vi "SHAPE_readTrainingData.vi"(8 "error in (no error)":errorcluster, 9 "ControlRefs":T1, 10 "NumberOfChannels":i32, 11 "BandGlobalOpt in":refnum<class "Shapelets Search GA.lvclass">) -> (0 "error out":errorcluster, 2 "TimeSeriesLength":i32, 3 "BandGlobalOpt out":refnum<class "Shapelets Search GA.lvclass">)   [LabVIEW 2016, in "Shapelets Search (GA).lvlib" / "Shapelets Search GA.lvclass"]
uses:
  Shapelets Search GA.lvclass
  Shapelets Search GA.lvclass/Shapelets Search GA.ctl
  <vilib>/xml/Load XML File.vi
  <vilib>/xml/Close Reference(Node).vi
  _XML_EEG_Features/XML_EEG_Features.lvlib
  <vilib>/xml/NI_XML.lvlib
panel:
  # "This VI is a part of BCI Design library, http://www.ru-bci.org \nCopyright © 2020, Sotnikov Peter, All rights reserved. License: CC BY-NC 4.0"
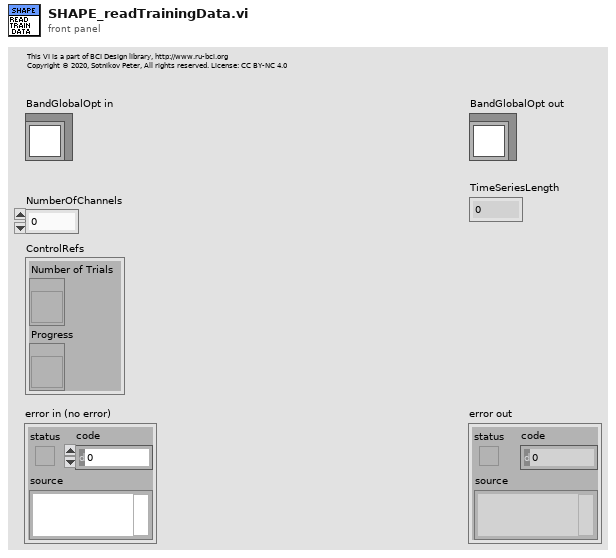
[diagram p1: front panel]
types:
  T1 = cluster{"Number of Trials":refnum<vi>, "Progress":refnum<vi>}
  T2 = typedef "XML_EEG_Features.lvlib/XML_FF_Header.ctl" = cluster{"NumberOfTrials":i32, "NumberOfClasses":i32, "FeatureVectorLength":i32, "FeatureExtractionMethod":string}
  T3 = typedef "XML_EEG_Features.lvlib/XML_FF_Trial.ctl" = cluster{"ClassLabel":string, "FeatureVector":dbl[]}
  T4 = cluster{"ClassLabel":string, "FeatureVector":dbl[][]}
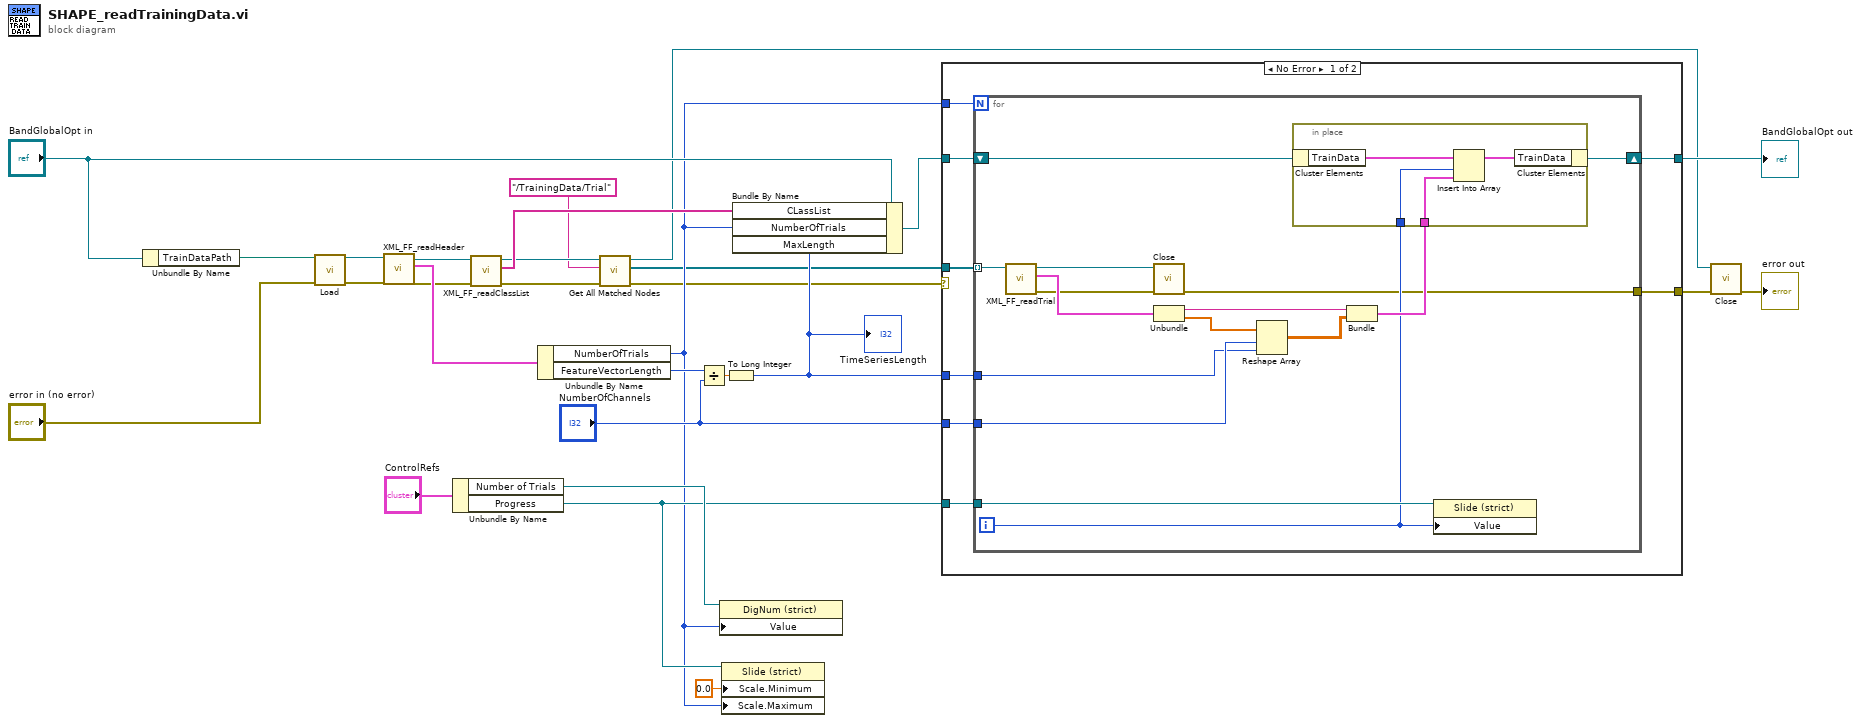
[diagram p0: block diagram]
diagram:
  n1 = Unbundle By Name("BandGlobalOpt in") -> ("TrainDataPath"=w28:path)
  n2 = call-poly <vilib>:"Load.vi"("path to XML document"=w28, "error in (no error)"="error in (no error)") -> ("DOM document out"=w25:refnum<k20>, "error out"=w26:errorcluster)  [unwired: 11 in, 1 out]
  n3 = call "XML_FF_readHeader.vi"("error in (no error)"=w26, "DOM document in"=w25) -> ("error out"=w12:errorcluster, "FF_Header out"=w24:T2, "DOM document out"=w13:refnum<k20>)  [unwired: 7 in]
  n4 = Unbundle By Name("ControlRefs") -> ("Number of Trials"=w16:refnum<vi>, "Progress"=w14:refnum<vi>)
  n5 = call "XML_FF_readClassList.vi"("error in (no error)"=w12, "DOM document in"=w13) -> ("error out"=w6:errorcluster, "CLassLabels out"=w9:string[], "DOM document out"=w4:refnum<k20>)  [unwired: 7 in]
  n6 = Unbundle By Name(w24) -> ("NumberOfTrials"=w8:i32, "FeatureVectorLength"=w23:i32)
  n7 = call <vilib>:"Get All Matched Nodes.vi"("error in (no error)"=w6, "XPath expression"="/TrainingData/Trial", "node in"=w4) -> ("error out"=w2:errorcluster, "node result array"=w5:refnum<k20>[], "node out"=w1:refnum<k20>)  [unwired: 6 in]
  n8 = Divide(x=w23, y="NumberOfChannels") -> (x/y=w18:dbl)
  n9 = property class="DigNum (strict)"(reference=w16, "Value"=w8) -> ()  [unwired: 1 in, 2 out]
  n10 = property class="Slide (strict)"(reference=w14, "Scale.Minimum"=0.0 ("Data Entry Limits:Minimum"), "Scale.Maximum"=w8) -> ()  [unwired: 1 in, 2 out]
  n11 = To Long Integer(number=w18) -> (32bit integer=w7:i32)
  "TimeSeriesLength" <- w7
  n12 = Bundle By Name(cluster="BandGlobalOpt in", "CLassList"=w9, "NumberOfTrials"=w8, "MaxLength"=w7) -> (w10:refnum<class "Shapelets Search GA.lvclass">)
  n13 = case shown="No Error" w2 {
    selector: w2 -> [_ w56]
    tunnel: w5 -> [w35 _]
    tunnel: w8 -> [w36 _]
    tunnel: w10 -> [w34 w57]
    tunnel: "NumberOfChannels" -> [w33 _]
    tunnel: w7 -> [w32 _]
    tunnel: [w31 w57] -> w21
    tunnel: [w30 w56] -> w20
    tunnel: w14 -> [w29 _]
    frame No Error {
      n14 = for {
        N: w36 -> [_]
        tunnel: w35 -> [w51] mode=indexing
        shift-right: [w49] -> w31
        shift-left: w34 -> [w50]
        tunnel: w33 -> [w46]
        tunnel: w32 -> [w45]
        tunnel: [w37] -> w30
        tunnel: w29 -> [w41]
        i -> [w40]
        n15 = call "XML_FF_readTrial.vi"("DOM document in"=w51) -> ("error out"=w38:errorcluster, "Trial out"=w48:T3, "DOM document out"=w39:refnum<k20>)  [unwired: 8 in]
        n16 = call-poly <vilib>:"Close.vi"("error in (no error)"=w38, "node"=w39) -> ("error out"=w37:errorcluster)  [unwired: 7 in]
        n17 = Unbundle(w48) -> ("ClassLabel"=w44:string, "FeatureVector"=w47:dbl[])
        n18 = Reshape Array(w47, w46, w45) -> (w43:dbl[][])
        n19 = Bundle("ClassLabel"=w44, "FeatureVector"=w43) -> (w42:T4)  [unwired: 1 in]
        n20 = in-place {
          in-place-border: w42 -> [w53]
          in-place-border: w40 -> [w52]
          n21 = in-place-cluster #1(w50) -> ("TrainData"=w55:cluster{"ClassLabel":string, "Trial":dbl[][]}[])
          n22 = Insert Into Array(array=w55, index=w52, new element=w53) -> (w54:cluster{"ClassLabel":string, "Trial":dbl[][]}[])
          n23 = in-place-cluster #1("TrainData"=w54) -> (w49:refnum<class "Shapelets Search GA.lvclass">)
        }
        n24 = property class="Slide (strict)"(reference=w41, "Value"=w40) -> ()  [unwired: 1 in, 2 out]
      }
    }
    frame Error {
    }
  }
  "BandGlobalOpt out" <- w21
  n25 = call-poly <vilib>:"Close.vi"("error in (no error)"=w20, "node"=w1) -> ("error out"=→"error out":errorcluster)  [unwired: 7 in]
